vi "CheckActors.vi"(10 "Actors":refnum<class "Actor.lvclass">[](array[class])) -> (2 "Error":errorcluster)   [LabVIEW 2020, in "jettl.lvlib"]
uses:
  jettl.lvlib
  Actor/Actor.lvclass
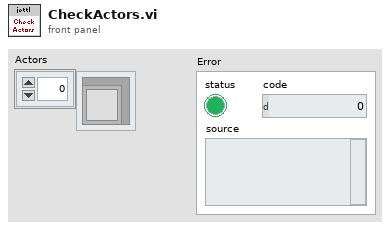
[diagram p1: front panel]
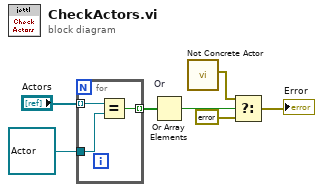
[diagram p0: block diagram]
diagram:
  n1 = for {
    tunnel: "Actors" -> [w9] mode=indexing
    tunnel: [w10] -> w2 mode=indexing
    tunnel: refnum<class "Actor.lvclass"> refnum ("jettl.lvlib:Actor.lvclass") -> [w8]
    n2 = Equal?(x=w9, y=w8) -> (x = y?=w10:bool)
  }
  n3 = Or Array Elements "Or"(Boolean array=w2) -> (logical OR=w6:bool)
  n4 = call "Not Concrete Actor.vi"() -> ("Error"=w7:errorcluster)  [unwired: 11 in]
  n5 = Select(t=w7, s=w6, f=errorcluster {"status"=FALSE, "code"=0, "source"=""}) -> (s? t:f=→"Error":errorcluster)
